vi "Assign XYZ Ramping.vi"(5 "Ramp Time [sec]":dbl=3.0, 6 "Vac Digital Cmd":i8, 7 "Robot In":i32, 8 "error in":errorcluster, 9 "Destination Posit Array [mm]":dbl[](array[numeric])=[0.0, 0.0, -3.0, 0.0], 11 "FPGA VI Reference In":refnum<k20>) -> (0 "error out":errorcluster, 3 "FPGA VI Reference Out":refnum<k20>)   [LabVIEW 2016]
uses:
  <vilib>/Analysis/1siggen.llb/Ramp Pattern by Samples.vi
  Subsystems/Global Variables.vi
  <vilib>/Analysis/NI_AALBase.lvlib
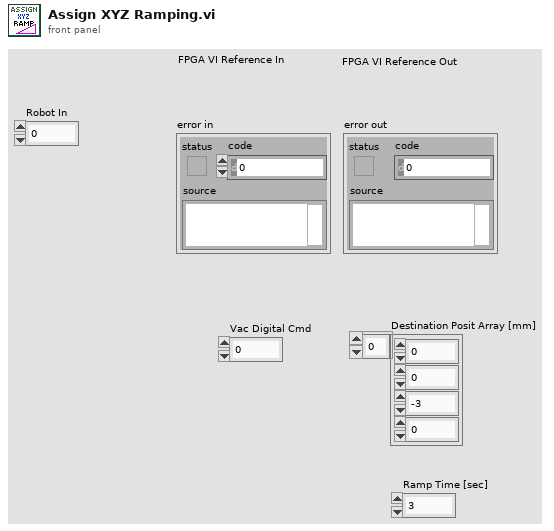
[diagram p1: front panel]
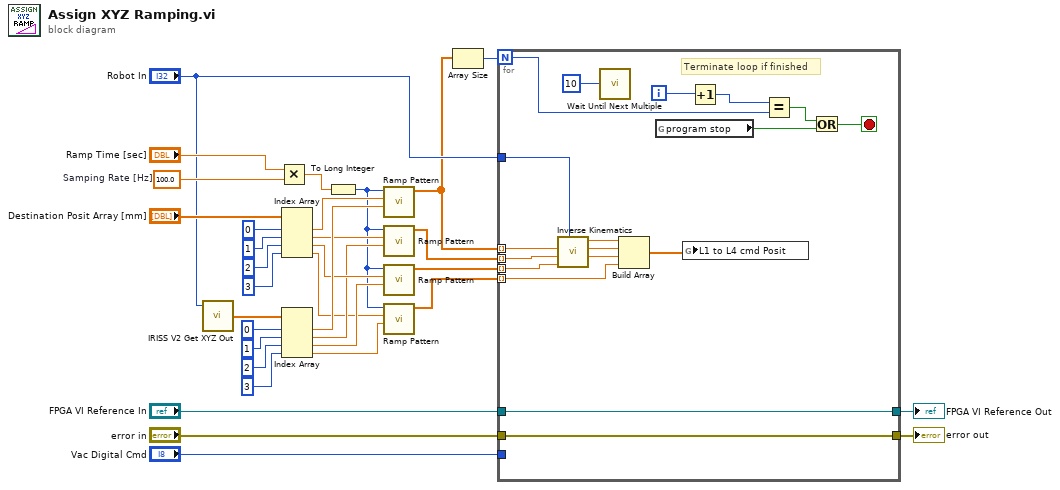
[diagram p0: block diagram]
diagram:
  w23 = 100.0  # Samping Rate [Hz]
  n1 = call "IRISS V2 Get XYZ Out.vi"("Left or Right Arm"="Robot In") -> ("XYZ Out Posit"=w5:dbl[])  [unwired: 3 in, 1 out]
  n2 = Multiply(x="Ramp Time [sec]", y=w23) -> (x*y=w14:dbl)
  n3 = Index Array(array="Destination Posit Array [mm]", index #1=0 ("index"), index #2=1 ("index"), index #3=2 ("index"), index #4=3 ("index")) -> (element #1=w21:dbl, element #2=w20:dbl, element #3=w19:dbl, element #4=w15:dbl)
  n4 = Index Array(array=w5, index #1=0 ("index"), index #2=1 ("index"), index #3=2 ("index"), index #4=3 ("index")) -> (element #1=w22:dbl, element #2=w18:dbl, element #3=w17:dbl, element #4=w16:dbl)
  n5 = To Long Integer(number=w14) -> (32bit integer=w4:i32)
  n6 = call-poly <vilib>:"Ramp Pattern.vi"("start"=w22, "end"=w21, "samples"=w4) -> ("Ramp Pattern"=w3:dbl[])  [unwired: 7 in, 1 out]
  n7 = call-poly <vilib>:"Ramp Pattern.vi"("start"=w18, "end"=w20, "samples"=w4) -> ("Ramp Pattern"=w13:dbl[])  [unwired: 7 in, 1 out]
  n8 = call-poly <vilib>:"Ramp Pattern.vi"("start"=w17, "end"=w19, "samples"=w4) -> ("Ramp Pattern"=w12:dbl[])  [unwired: 7 in, 1 out]
  n9 = call-poly <vilib>:"Ramp Pattern.vi"("start"=w16, "end"=w15, "samples"=w4) -> ("Ramp Pattern"=w11:dbl[])  [unwired: 7 in, 1 out]
  n10 = Array Size(array=w3) -> (size(s)=w2:i32)
  n11 = for {
    N: w2 -> [w42]
    tunnel: w3 -> [w40] mode=indexing
    tunnel: w13 -> [w39] mode=indexing
    tunnel: w12 -> [w50] mode=indexing
    tunnel: w11 -> [w38] mode=indexing
    tunnel: "Vac Digital Cmd" -> [_]
    tunnel: "Robot In" -> [w37]
    tunnel: "FPGA VI Reference In" -> [w35]
    tunnel: [w35] -> w8
    tunnel: "error in" -> [w34]
    tunnel: [w34] -> w10
    i -> [w44]
    stop <- w45 stop-if-true
    # "Terminate loop if finished"
    n12 = call "Inverse Kinematics.vi"("armID"=w37, "z"=w50, "y"=w39, "x"=w40) -> ("j3"=w47:dbl, "j2"=w48:dbl, "j1"=w49:dbl)  [unwired: 4 in, 1 out]
    n13 = call "Wait Until Next Multiple"("Count(mSec)"=u32 10) -> ()  [unwired: 1 out]
    n14 = Build Array(w49, w48, w47, w38) -> (w36:dbl[])
    n15 = global read "Global Variables.vi" "program stop"() -> (w46:bool)
    n16 = global write "Global Variables.vi" "L1 to L4 cmd Posit"(w36) -> ()
    n17 = Increment(x=w44) -> (x+1=w43:i32)
    n18 = Equal?(x=w43, y=w42) -> (x = y?=w41:bool)
    n19 = Or(x=w41, y=w46) -> (x .or. y?=w45:bool)
  }
  "error out" <- w10
  "FPGA VI Reference Out" <- w8
